vi "SECoP_dataPutEnumeration.vi"(4 "enumeration_name":string, 6 "Enumval":i64, 7 "Position":u32, 8 "error in (no error)":errorcluster, 9 "Index":u32, 10 "SECoP_dataPtr in":T1 {"ptr64" format="%.0x"; "ptr32" format="%.0x"}, 11 "DLL path (in)":T2) -> (0 "error out":errorcluster, 3 "DLL path (out)":T2)   [LabVIEW 2023, in "SECoP.lvlib"]
doc: "Call <b>\"SECoP_dataGetEnumeration.vi\"</b> to extend the enumeration of a complex data type with a new pair of numeric value with name.\n\n<b>DLL path</b> input and output of cluster from \"SECoP-Initialize.vi\"\n<b>SECoP_dataPtr</b> data to access\n<b>Position</b> points to a virtual flattened entry of the data type; for a simple enumeration use 0\n<b>Index</b> index of the enumeration (starting with 0 to \"SECoP_dataGetEnumerationCount.vi\" - 1)\n<b>EnumVal</b> new unique integer value of enumeration\n<b>enumeration_name</b> new unique name of the enumeration"
uses:
  SECoP.lvlib
  SECoP-libraries.ctl
  SECoP-data.ctl
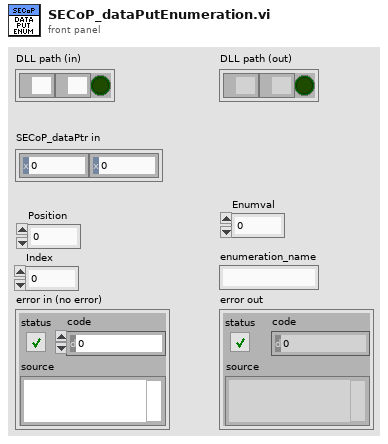
[diagram p1: front panel]
types:
  T1 = typedef "SECoP.lvlib/SECoP-data.ctl" = cluster{"ptr32":u32, "ptr64":u64}
  T2 = typedef "SECoP.lvlib/SECoP-libraries.ctl" = cluster{"serverDLL":path, "variantDLL":path, "cleanup_mode":bool}
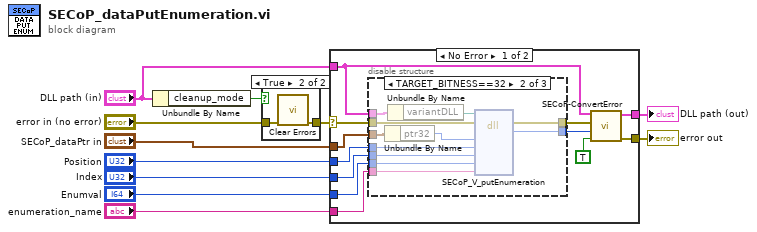
[diagram p0: block diagram]
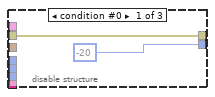
[diagram p3: hidden frame]
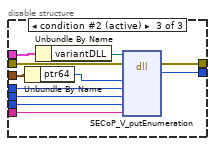
[diagram p4: hidden frame]
diagram:
  n1 = Unbundle By Name("DLL path (in)") -> ("cleanup_mode"=w8:bool)
  n2 = case shown="True" w8 {
    tunnel: "error in (no error)" -> [w12 w14]
    tunnel: [w12 w13] -> w6
    frame False {
    }
    frame True {
      n3 = call <vilib>:"Clear Errors.vi"("error in (no error)"=w14) -> ("error out"=w13:errorcluster)  [unwired: 5 in, 1 out]
    }
  }
  n4 = case shown="No Error" w6 {
    selector: w6 -> [w26 w51]
    tunnel: "DLL path (in)" -> [w15 w52]
    tunnel: [w17 w52] -> w10
    tunnel: [w16 w51] -> w9
    tunnel: "Position" -> [w25 _]
    tunnel: "Index" -> [w24 _]
    tunnel: "SECoP_dataPtr in" -> [w23 _]
    tunnel: "Enumval" -> [w22 _]
    tunnel: "enumeration_name" -> [w21 _]
    frame No Error {
      n5 = disable-structure shown="TARGET_BITNESS==32" {
        disable-tunnel: w26 -> [w28 w39 w50]
        disable-tunnel: w15 -> [_ w38 w49]
        disable-tunnel: w25 -> [_ w37 w48]
        disable-tunnel: w24 -> [_ w36 w47]
        disable-tunnel: [w28 w35 w46] -> w18
        disable-tunnel: [-20 w30 w41] -> w19
        disable-tunnel: w23 -> [_ w34 w45]
        disable-tunnel: w22 -> [_ w32 w43]
        disable-tunnel: w21 -> [_ w31 w42]
        frame condition #0 {
        }
        frame condition #1 {
          n6 = Unbundle By Name(w34) -> ("ptr32"=w33:u32)
          n7 = Unbundle By Name(w38) -> ("variantDLL"=w29:path)
          n8 = dll-call lib="Z:/Praktische_Aufgaben/SECoP-LabVIEW2015/32bit/SECoP32.dll" fn="SECoP_V_putEnumeration"(path in=w29, error in=w39, "pData"=w33, "uPosition"=w37, "uIndex"=w36, "llEnumVal"=w32, "szEnumName"=w31) -> (error out=w35:errorcluster, "return type"=w30:i32)  [unwired: 6 in, 1 out]
        }
        frame condition #2 (active) {
          n9 = Unbundle By Name(w45) -> ("ptr64"=w44:u64)
          n10 = Unbundle By Name(w49) -> ("variantDLL"=w40:path)
          n11 = dll-call lib="Z:/Praktische_Aufgaben/SECoP-LabVIEW2015/32bit/SECoP32.dll" fn="SECoP_V_putEnumeration"(path in=w40, error in=w50, "pData"=w44, "uPosition"=w48, "uIndex"=w47, "llEnumVal"=w43, "szEnumName"=w42) -> (error out=w46:errorcluster, "return type"=w41:i32)  [unwired: 6 in, 1 out]
        }
      }
      n12 = call "SECoP-ConvertError.vi"("return is boolean"=TRUE, "return code"=w19, "error in (no error)"=w18, "DLL path (in)"=w15) -> ("error out"=w16:errorcluster, "DLL path (out)"=w17:T2)  [unwired: 6 in]
    }
    frame Error {
    }
  }
  "DLL path (out)" <- w10
  "error out" <- w9
